vi "calculateFaultIndicatorsTest.vi"(5 "AnalysisSettings":T1={"Fault Thresholds"={"Parameters labels"=[], "Parameters thresholds"=[], "Freqs and thresholds"=[], "Orders and thresholds"=[]}, "Analysis series name"="Analiza", "Save data analysis?"=TRUE, "F-Band Size"=20, "OrderAnalysis?"=TRUE, "Accelerometer"=enum."MMA7351", "fs [Hz]"=4000.0, "Pulse per revolution"=1, "FFT-Parameters"={"averaging mode"=enum."No averaging", "weighting mode"=enum."Linear", "number of averages"=0}, "O-WindowPowerSpectrum"=0, "O-SpectrumAveraging"=enum."No averaging", "O-MaxOrder"=0.0, "O-Resolution"=0.0, "O-BandSize"=0.0, "FrameLength [s]"=1.0}, 7 "fs [Hz]":dbl=4000.0, 8 "ErrorIn":errorcluster, 9 "spectrum info":T5[](array[typedef])=[{"channel name"="Channel0", "description"="", "x-axis units"=4, "spectral info"={"spectrum type"=enum."Power [Magnitude^2]", "linear/dB"=enum."linear", "window"=0, "window size"=2147483647, "FFT size"=2147483647}, "engineering units"=0, "custom label"="EU", "dB reference [EU]"=1.0, "peak units"=enum."rms", "weighting filter"=0, "spectral density?"=FALSE, "unit label"="EU^2 rms|SV Units|dB rms ref 1,0E+0 EU", "spectrum skewed?"=FALSE, "complimentary spectrum units"=enum."none"}, {"channel name"="Channel1", "description"="", "x-axis units"=4, "spectral info"={"spectrum type"=enum."Power [Magnitude^2]", "linear/dB"=enum."linear", "window"=0, "window size"=2147483647, "FFT size"=2147483647}, "engineering units"=0, "custom label"="EU", "dB reference [EU]"=1.0, "peak units"=enum."rms", "weighting filter"=0, "spectral density?"=FALSE, "unit label"="EU^2 rms|SV Units|dB rms ref 1,0E+0 EU", "spectrum skewed?"=FALSE, "complimentary spectrum units"=enum."none"}, {"channel name"="Channel2", "description"="", "x-axis units"=4, "spectral info"={"spectrum type"=enum."Power [Magnitude^2]", "linear/dB"=enum."linear", "window"=0, "window size"=2147483647, "FFT size"=2147483647}, "engineering units"=0, "custom label"="EU", "dB reference [EU]"=1.0, "peak units"=enum."rms", "weighting filter"=0, "spectral density?"=FALSE, "unit label"="EU^2 rms|SV Units|dB rms ref 1,0E+0 EU", "spectrum skewed?"=FALSE, "complimentary spectrum units"=enum."none"}] {"x-axis units" items=["Time (s)"=0, "Frequency-CB (Hz)"=1, "Frequency-CPB (Hz)"=1248, "Frequency-Arbitrary (Hz)"=2357, "Quefrency (s)"=2, "Revolutions (rev)"=3, "Order"=4, "Speed (RPM)"=11, "Speed (rad/s)"=21, "Index"=65535]; "weighting filter" items=["Linear", "A-weighting", "B-weighting", "C-weighting", "ITU-R 468-4", "Dolby", "CCITT", "C-message", "Wb", "Wc", "Wd", "We", "Wf", "Wh", "Wj", "Wk", "Wm", "AES17 20 kHz lowpass", "AES17 40 kHz lowpass", "AES17 20 kHz highpass", "AES17 40 kHz highpass"]; "dB reference [EU]" format="%.2f"; "engineering units" items=["custom..."=0, "V"=1, "A"=21, "C"=30, "pC"=31, "s"=32, "-"=29, "Pa"=2, "N"=20, "g"=3, "m/s^2"=4, "m/s"=5, "m"=6, "mm/s"=12, "mm"=13, "micron/s"=14, "micron"=15, "in/s^2"=7, "in/s"=8, "in"=9, "mil/s"=10, "mil"=11, "rad/s^2"=16, "rad/s"=17, "rad"=18, "deg/s^2"=26, "deg/s"=27, "deg"=28, "RPM"=22, "cycle/s^2"=23, "Hz"=24, "cycle"=25, "strain"=19]; "spectral info"."window" items=["None "=0, "Hanning"=1, "Hamming"=2, "Blackman-Harris"=3, "Exact Blackman"=4, "Blackman"=5, "Flat Top"=6, "4 Term B-Harris "=7, "7 Term B-Harris"=8, "Low Sidelobe"=9, "Force - Exponential"=10, "Gaussian"=62]}, 10 "order power spectra":T12(array[cluster]) {"order 0" format="%.2p"; "delta order" format="%.2p"; "magnitude" format="%.2f"}, 11 "AccelerationDataFrames":T14={"AccelerationData"=[{"t0"=timestamp(2.0995 s since 1904-01-01), "dt"=0.00025, "Y"=array[4200 elements]}, {"t0"=timestamp(2.0995 s since 1904-01-01), "dt"=0.00025, "Y"=array[4200 elements]}, {"t0"=timestamp(2.0995 s since 1904-01-01), "dt"=0.00025, "Y"=array[4200 elements]}], "Amplitudes"=[{"f0"=0.0, "df"=0.9523809523809523, "real part"=array[2100 elements]}, {"f0"=0.0, "df"=0.9523809523809523, "real part"=array[2100 elements]}, {"f0"=0.0, "df"=0.9523809523809523, "real part"=array[2100 elements]}], "Phases"=[{"f0"=0.0, "df"=0.9523809523809523, "imaginary part"=array[2100 elements]}, {"f0"=0.0, "df"=0.9523809523809523, "imaginary part"=array[2100 elements]}, {"f0"=0.0, "df"=0.9523809523809523, "imaginary part"=array[2100 elements]}]}) -> (0 "ErrorOut":errorcluster, 2 "Orders and indicators":T11[](array[typedef]), 3 "Fault Indicators":T13)   [LabVIEW 2019]
uses:
  MobileAnalyzer/mainVIs/analyzeAccelerationDataVIs/AccelerationDataFrames.ctl
  MobileAnalyzer/mainVIs/analyzeAccelerationDataVIs/calculateFaultIndicatorsVIs/FaultIndicators.ctl
  MobileAnalyzer/mainVIs/analyzeAccelerationDataVIs/OrderAndIndicators.ctl
  <vilib>/addons/_NISVFA/_Shared subVIs/Controls/svc_Spectrum Info.ctl
  <vilib>/addons/_NISVFA/_Shared subVIs/Controls/svc_X-Axis Units.ctl
  <vilib>/addons/_NISVFA/_Shared subVIs/Controls/svc_Spectrum Type.ctl
  <vilib>/addons/_NISVFA/_Shared subVIs/Controls/svc_Engineering Units Text Ring.ctl
  <vilib>/addons/_NISVFA/_Shared subVIs/Controls/svc_Weighting Filter Text Ring.ctl
  <vilib>/addons/_NISVFA/_Shared subVIs/Controls/svc_Complimentary Spectrum Units.ctl
  VibrationDiagnosisDesktopApp/mainVIs/DialogsVIs/AnalysisSettings.ctl
  MobileAnalyzer/mainVIs/analyzeAccelerationDataVIs/calculateFaultIndicatorsVIs/Thresholds.ctl
  MobileAnalyzer/mainVIs/analyzeAccelerationDataVIs/calculateFaultIndicatorsVIs/FaultParameter.ctl
  MobileAnalyzer/mainVIs/aquireAccelerationDataVIs/Accelerometer.ctl
  <vilib>/Analysis/5stat.llb/RMS (DBL).vi
  <vilib>/addons/_NISVFA/_Spectrum Processing/SVFA Power in Band (N Ch).vi
  <vilib>/addons/_NISVFA/_Spectrum Processing/SVFA Power in Band (1 Ch).vi
  <vilib>/addons/_NISVFA/_Spectrum Processing/SVFA Get Spectrum Subset.vi
  <vilib>/addons/_NISVFA/_Spectrum Processing/SVFA Get Spectrum Subset (1 Ch).vi
  <vilib>/addons/_NISVFA/_Shared subVIs/Common/svc_Spectrum Units.vi
  <vilib>/addons/_NISVFA/_Spectrum Processing/SVFA Unit Conversion.vi
  <vilib>/addons/_NISVFA/_Spectrum Processing/SVFA Unit Conversion (1 Ch).vi
  <vilib>/dlg_ctls.llb/Space Constant.vi
  <vilib>/addons/_NISVFA/_Spectrum Processing/subVIs/svfa_Conversion Utility (spectrum info).vi
  <vilib>/addons/_NISVFA/_Spectrum Processing/subVIs/svfa_Peak to RMS to Peak2Peak.vi
  <vilib>/addons/_NISVFA/_Spectrum Processing/subVIs/svfa_Mag to Mag2.vi
  <vilib>/addons/_NISVFA/_Spectrum Processing/subVIs/svfa_Linear to dB.vi
  <vilib>/addons/_NISVFA/_Spectrum Processing/subVIs/svfa_dBrefA to dBrefB.vi
  <vilib>/addons/_NISVFA/_Spectrum Processing/subVIs/svfa_Spectrum to Spectral Density.vi
  <vilib>/measure/madcrms.llb/Basic Averaged DC-RMS for 1 Chan.vi
  <vilib>/addons/Digital Filter Design/Process.llb/DFD Filtering (Wfm NChan).vi
  <vilib>/measure/madcrms.llb/Basic Averaged DC-RMS for N Chan.vi
  <vilib>/addons/_NISVFA/_Shared subVIs/Common/svc_Format Value (DBL).vi
  <vilib>/addons/_NISVFA/_Shared subVIs/Common/svc_Engineering Units to Unit Label.vi
  <vilib>/addons/_NISVFA/_Shared subVIs/Common/svc_Surround NonAlpha String with Parentheses.vi
  <vilib>/addons/_NISVFA/_Shared subVIs/Common/svc_Get Weighting Enum and Labels.vi
  <vilib>/addons/_NISVFA/_Shared subVIs/Common/svc_Check Frequency Range in Spectrum.vi
  <vilib>/addons/_NISVFA/_Shared subVIs/Common/svc_Caller VI Returned in Error Source.vi
  <vilib>/addons/_NISVFA/_Shared subVIs/Common/svc_Convert Frequency to Frequency String.vi
  <vilib>/addons/_NISVFA/_Shared subVIs/Common/svc_Build Unit Label for Frequency Range.vi
  <vilib>/addons/_NISVFA/_Shared subVIs/Common/svc_Window Parameters.vi
  <vilib>/addons/_NISVFA/_Spectrum Processing/subVIs/svfa_Spectrum Info Window to windowTd Type Def.vi
  <vilib>/gmath/NI_Gmath.lvlib
  <vilib>/measure/NI_MAPro.lvlib
  <vilib>/Analysis/NI_AALPro.lvlib
  <vilib>/addons/Digital Filter Design/NI_DigFilterLicensed.lvlib
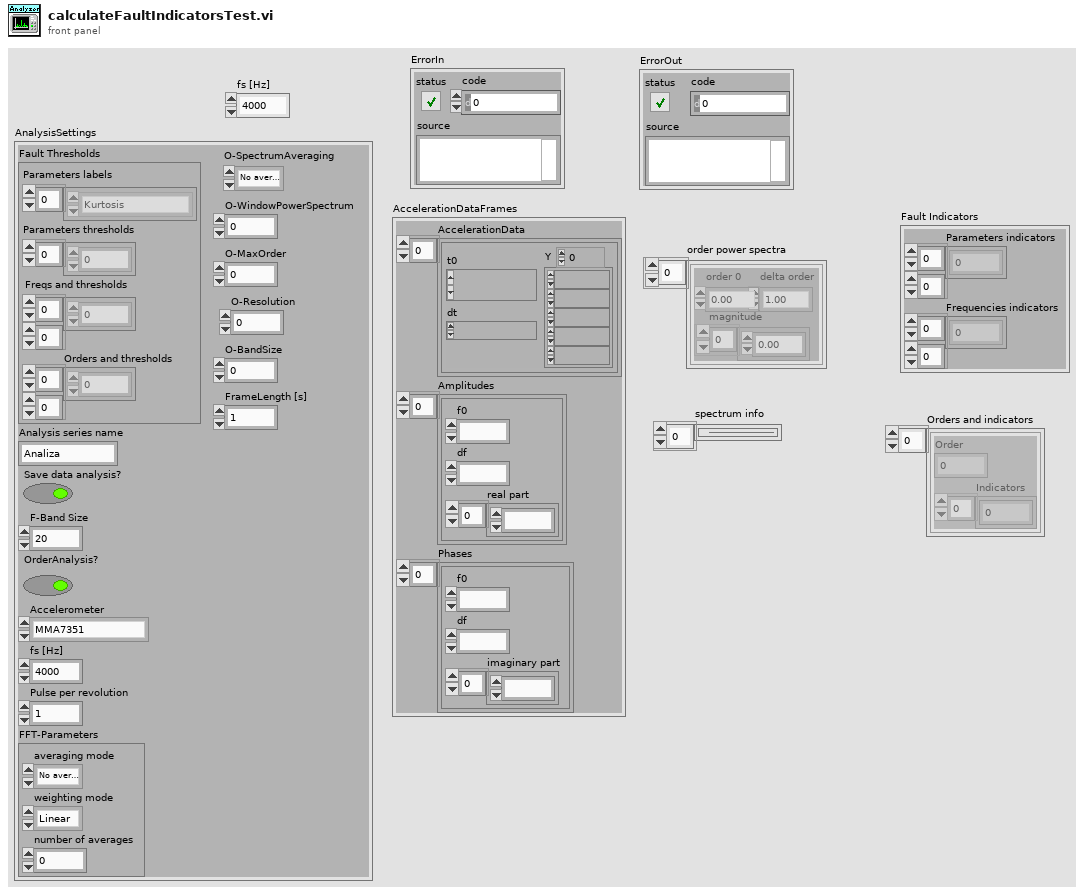
[diagram p1: front panel]
types:
  T1 = typedef "AnalysisSettings.ctl" = cluster{"Fault Thresholds":T2, "Analysis series name":string, "Save data analysis?":bool, "F-Band Size":i32, "OrderAnalysis?":bool, "Accelerometer":T4, "fs [Hz]":dbl, "Pulse per revolution":u16, "FFT-Parameters":cluster{"averaging mode":enum16{"No averaging", "Vector averaging", "RMS averaging", "Peak hold"}, "weighting mode":enum16{"Linear", "Exponential"}, "number of averages":u32}, "O-WindowPowerSpectrum":u32, "O-SpectrumAveraging":enum16{"No averaging", "Vector averaging", "RMS averaging", "Peak hold"}, "O-MaxOrder":dbl, "O-Resolution":dbl, "O-BandSize":dbl, "FrameLength [s]":dbl}
  T2 = typedef "Thresholds.ctl" = cluster{"Parameters labels":T3[], "Parameters thresholds":dbl[], "Freqs and thresholds":dbl[][], "Orders and thresholds":dbl[][]}
  T3 = typedef "FaultParameter.ctl" = enum16{"Kurtosis", "RMS", "Crest factor"}
  T4 = typedef "Accelerometer.ctl" = enum16{"None", "MPU6050", "MMA7351"}
  T5 = typedef "svc_Spectrum Info.ctl" = cluster{"channel name":string, "description":string, "x-axis units":T6, "spectral info":cluster{"spectrum type":T7, "linear/dB":enum16{"linear", "dB"}, "window":u16, "window size":i32, "FFT size":i32}, "engineering units":T8, "custom label":string, "dB reference [EU]":dbl, "peak units":enum16{"rms", "peak", "peak-peak"}, "weighting filter":T9, "spectral density?":bool, "unit label":string, "spectrum skewed?":bool, "complimentary spectrum units":T10}
  T6 = typedef "svc_X-Axis Units.ctl" = u16
  T7 = typedef "svc_Spectrum Type.ctl" = enum16{"FFT Spectrum [complex]", "Amplitude [Magnitude]", "Power [Magnitude^2]", "Cross Spectrum [complex]", "Frequency Response [Complex]"}
  T8 = typedef "svc_Engineering Units Text Ring.ctl" = u16
  T9 = typedef "svc_Weighting Filter Text Ring.ctl" = u16
  T10 = typedef "svc_Complimentary Spectrum Units.ctl" = enum16{"none", "radians", "degrees", "cycles", "imaginary"}
  T11 = typedef "OrderAndIndicators.ctl" = cluster{"Order":dbl, "Indicators":dbl[]}
  T12 = cluster{"order 0":dbl, "delta order":dbl, "magnitude":dbl[]}[]
  T13 = typedef "FaultIndicators.ctl" = cluster{"Parameters indicators":dbl[][], "Frequencies indicators":dbl[][]}
  T14 = typedef "AccelerationDataFrames.ctl" = cluster{"AccelerationData":waveform(dbl)[], "Amplitudes":cluster{"f0":dbl, "df":dbl, "real part":dbl[]}[], "Phases":cluster{"f0":dbl, "df":dbl, "imaginary part":dbl[]}[]}
  T15 = enum16{"Lowpass", "Highpass", "Bandpass", "Bandstop"}
  T16 = typedef "NI_DigFilterLicensed.lvlib/DFD Filter Obj.ctl" = cluster{"mSRate_Fs":dbl, "mSRate_Version":string, "mSRate_Comments":string, "mSRate_OrgCoef":T17, "mSRate_CurCoef":T17, "mSRate_Quantized?":bool, "mSRate_QCoef":T17, "mSRate_QSettings":T19[], "mSRate_Order":i32, "mSRate_Scaling":cluster{"mSRate_ScaleByPowerOf2?":bool, "mSRate_ScaleType":T21}}
  T17 = typedef "NI_DigFilterLicensed.lvlib/DFD Filter Coef.ctl" = cluster{"type":T18, "gain":dbl, "coef a (k)":dbl[], "coef b (v)":dbl[]}
  T18 = typedef "NI_DigFilterLicensed.lvlib/DFD Filter Structure Type Selector.ctl" = enum16{"Undefined", "FIR Direct Form", "FIR Direct Form Transposed", "FIR Symmetric", "FIR Antisymmetric", "IIR Direct Form I", "IIR Direct Form I Transposed", "IIR Direct Form II", "IIR Direct Form II Transposed", "IIR Cascaded Second Order Sections Form I", "IIR Cascaded Second Order Sections Form I Transposed", "IIR Cascaded Second Order Sections Form II", "IIR Cascaded Second Order Sections Form II Transposed", "Lattice Allpass (basic sections)", "Lattice Allpass (one multiplier sections)", "Lattice Allpass (normalized sections)", "Lattice AR (basic sections)", "Lattice AR (one multiplier sections)", "Lattice AR (normalized sections)", "Lattice MA (minimum phase)", "Lattice MA (maximum phase)", "Lattice ARMA (basic sections)", "Lattice ARMA (one multiplier sections)", "Lattice ARMA (normalized sections)"}
  T19 = typedef "NI_DigFilterLicensed.lvlib/dfd_Internal Quantization Settings.ctl" = cluster{"source":T20, "wl":i16, "iwl":i16, "overflow mode":enum16{"Saturation", "Wrap"}, "rounding mode":enum16{"Nearest", "Truncation"}, "signed?":bool}
  T20 = typedef "NI_DigFilterLicensed.lvlib/dfd_Internal Quantization Srcs.ctl" = u16
  T21 = typedef "NI_DigFilterLicensed.lvlib/DFD Coef Norm Type.ctl" = enum16{"No Norm", "Time Domain 1-Norm", "Time Domain 2-Norm", "Time Domain Inf-Norm"}
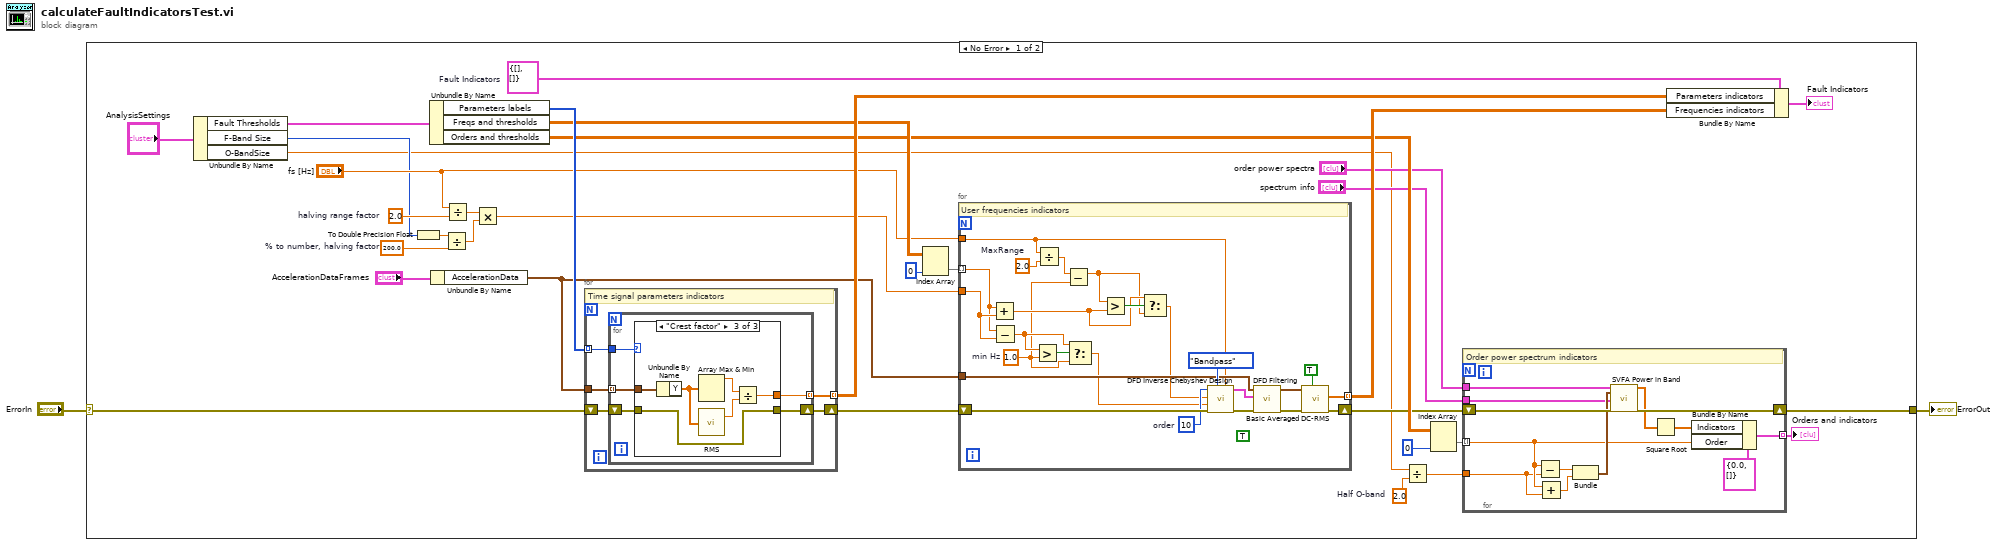
[diagram p0: block diagram]
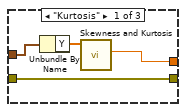
[diagram p2: hidden frame]
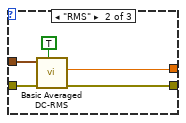
[diagram p3: hidden frame]
diagram:
  n1 = case shown="No Error" "ErrorIn" {
    selector: "ErrorIn" -> [w32 w98]
    tunnel: [w14 w98] -> w1
    frame No Error {
      w7 = 2.0  # Half O-band
      w13 = 2.0  # halving range factor
      w21 = 200.0  # % to number, halving factor
      w35 = T13 {"Parameters indicators"=[], "Frequencies indicators"=[]}  # Fault Indicators
      n2 = Unbundle By Name("AnalysisSettings") -> ("Fault Thresholds"=w5:T2, "F-Band Size"=w4:i32, "O-BandSize"=w3:dbl)
      n3 = To Double Precision Float(number=w4) -> (double precision float=w22:dbl)
      n4 = Unbundle By Name(w5) -> ("Parameters labels"=w33:T3[], "Freqs and thresholds"=w29:dbl[][], "Orders and thresholds"=w19:dbl[][])
      n5 = Unbundle By Name("AccelerationDataFrames") -> ("AccelerationData"=w23:waveform(dbl)[])
      n6 = Divide(x=w22, y=w21) -> (x/y=w11:dbl)
      n7 = Divide(x="fs [Hz]", y=w13) -> (x/y=w12:dbl)
      n8 = Multiply(x=w12, y=w11) -> (x*y=w10:dbl)
      n9 = for {
        tunnel: w23 -> [w77]
        tunnel: w33 -> [w76] mode=indexing
        shift-right: [w74] -> w30
        shift-left: w32 -> [w75]
        tunnel: [w73] -> w31 mode=indexing
        # "Time signal parameters indicators"
        n10 = for {
          tunnel: w77 -> [w82] mode=indexing
          tunnel: [w81] -> w73 mode=indexing
          tunnel: w76 -> [w80]
          shift-right: [w78] -> w74
          shift-left: w75 -> [w79]
          n11 = case shown="\"Crest factor\"" w80 {
            tunnel: w82 -> [w86 w91 w92]
            tunnel: [w84 w87 w94] -> w81
            tunnel: w79 -> [w83 w89 w93]
            tunnel: [w83 w88 w93] -> w78
            frame "Kurtosis" {
              n12 = Unbundle By Name(w86) -> ("Y"=w85:dbl[])
              n13 = call <vilib>:"Skewness and Kurtosis.vi"("X"=w85) -> ("kurtosis"=w84:dbl)  [unwired: 8 in, 2 out]
            }
            frame "RMS" {
              n14 = call-poly <vilib>:"Basic Averaged DC-RMS.vi"("reset"=TRUE, "error in (no error)"=w89, "signal in"=w91) -> ("error out"=w88:errorcluster, "RMS value"=w87:dbl)  [unwired: 5 in, 2 out]
            }
            frame "Crest factor" {
              n15 = Unbundle By Name(w92) -> ("Y"=w97:dbl[])
              n16 = Array Max & Min(array=w97) -> (max value=w96:dbl)  [unwired: 3 out]
              n17 = call-poly <vilib>:"RMS.vi"("X"=w97) -> ("rms value"=w95:dbl)  [unwired: 1 out]
              n18 = Divide(x=w96, y=w95) -> (x/y=w94:dbl)
            }
          }
        }
      }
      n19 = Index Array(array=w29, index (col)=0 ("disabled index (col)")) -> (element=w27:dbl[])  [unwired: 1 in]
      n20 = for {
        shift-right: [w62] -> w16
        shift-left: w30 -> [w72]
        tunnel: w23 -> [w67]
        tunnel: w27 -> [w60] mode=indexing
        tunnel: [w63] -> w26 mode=indexing
        tunnel: "fs [Hz]" -> [w53]
        tunnel: w10 -> [w61]
        w49 = 1.0  # min Hz
        w59 = 2.0  # MaxRange
        (unwired) TRUE ("init/cont (init:F)")
        w70 = 10  # order
        # "User frequencies indicators"
        n21 = Add(x=w60, y=w61) -> (x+y=w52:dbl)
        n22 = Subtract(x=w60, y=w61) -> (x-y=w55:dbl)
        n23 = Greater?(x=w55, y=w49) -> (0:w56:bool)
        n24 = Divide(x=w53, y=w59) -> (x/y=w51:dbl)
        n25 = Subtract(x=w51, y=w49) -> (x-y=w50:dbl)
        n26 = Select(t=w55, s=w56, f=w49) -> (s? t:f=w54:dbl)
        n27 = Greater?(x=w50, y=w52) -> (0:w58:bool)
        n28 = Select(t=w52, s=w58, f=w50) -> (s? t:f=w57:dbl)
        n29 = call <vilib>:"DFD Inverse Chebyshev Design.vi"("fs [Hz]"=w53, "filter type"=T15."Bandpass", "error in (no error)"=w72, "low cutoff freq [Hz]"=w54, "high cutoff freq [Hz]"=w57, "order"=w70) -> ("error out"=w69:errorcluster, "filter out"=w68:T16)  [unwired: 4 in]
        n30 = call-poly <vilib>:"DFD Filtering.vi"("error in (no error)"=w69, "filter"=w68, "signal in"=w67) -> ("error out"=w65:errorcluster, "signal out"=w66:waveform(dbl)[])  [unwired: 7 in]
        n31 = call-poly <vilib>:"Basic Averaged DC-RMS.vi"("reset"=TRUE, "error in (no error)"=w65, "signals in"=w66) -> ("error out"=w62:errorcluster, "RMS values"=w63:dbl[])  [unwired: 5 in, 2 out]
      }
      n32 = Divide(x=w3, y=w7) -> (x/y=w8:dbl)
      n33 = Index Array(array=w19, index (col)=0 ("disabled index (col)")) -> (element=w24:dbl[])  [unwired: 1 in]
      n34 = for {
        shift-right: [w47] -> w14
        shift-left: w16 -> [w48]
        tunnel: w24 -> [w41] mode=indexing
        tunnel: [w42] -> w15 mode=indexing
        tunnel: "order power spectra" -> [w40]
        tunnel: "spectrum info" -> [w39]
        tunnel: w8 -> [w37]
        # "Order power spectrum indicators"
        n35 = Subtract(x=w41, y=w37) -> (x-y=w46:dbl)
        n36 = Add(x=w41, y=w37) -> (x+y=w45:dbl)
        n37 = Bundle(w46, w45) -> (w44:cluster{dbl, dbl})  [unwired: 1 in]
        n38 = call-poly <vilib>:"SVFA Power in Band.vi"("spectra"=w40, "range"=w44, "spectrum info"=w39, "error in (no error)"=w48) -> ("powers in band"=w38:dbl[], "error out"=w47:errorcluster)  [unwired: 13 in, 1 out]
        n39 = Square Root(x=w38) -> (sqrt(x)=w36:dbl[])
        n40 = Bundle By Name(cluster=T11 {"Order"=0.0, "Indicators"=[]} ("Order and indicators"), "Indicators"=w36, "Order"=w41) -> (w42:T11)
      }
      "Orders and indicators" <- w15
      n41 = Bundle By Name(cluster=w35, "Parameters indicators"=w31, "Frequencies indicators"=w26) -> (→"Fault Indicators":T13)
    }
    frame Error {
    }
  }
  "ErrorOut" <- w1
